vi "Reset.vi"(8 "error in (no error)":errorcluster, 11 "PWM in":refnum<class "LINX-PCA9685 PWM.lvclass">) -> (0 "error out":errorcluster, 3 "PWM out":refnum<class "LINX-PCA9685 PWM.lvclass">)   [LabVIEW 2020, in "LINX-PCA9685 PWM.lvclass"]
uses:
  LINX-PCA9685 PWM.lvclass
  LINX I2C/LINX I2C.lvclass
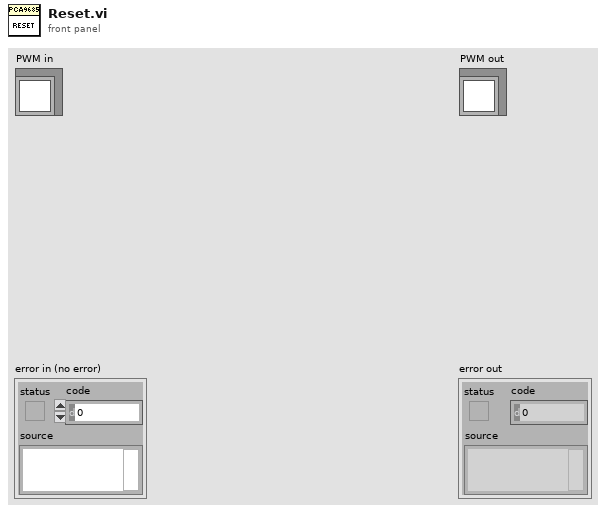
[diagram p1: front panel]
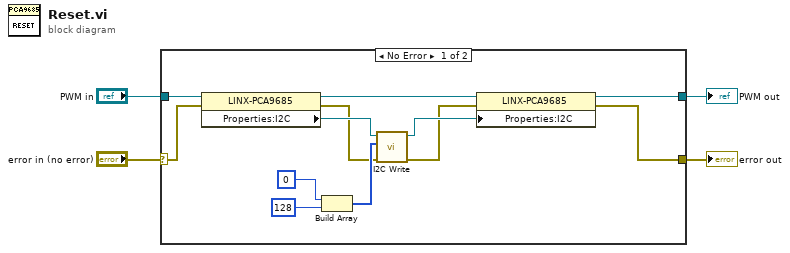
[diagram p0: block diagram]
diagram:
  n1 = case shown="No Error" "error in (no error)" {
    selector: "error in (no error)" -> [w6 w18]
    tunnel: [w7 w18] -> w3
    tunnel: [w9 w17] -> w1
    tunnel: "PWM in" -> [w13 w17]
    frame No Error {
      n2 = property class="LINX-PCA9685"(reference=w13, error in=w6) -> (reference out=w10:refnum<class "LINX-PCA9685 PWM.lvclass">, error out=w5:errorcluster, "Properties:I2C"=w12:refnum<class "LINX I2C.lvclass">)
      n3 = Build Array(u8 0 ("Address"), u8 128 ("Address")) -> (w16:u8[])
      n4 = call "I2C Write.vi"("error in (no error)"=w5, "Bytes to Write"=w16, "LINX I2C in"=w12) -> ("error out"=w8:errorcluster, "LINX I2C out"=w11:refnum<class "LINX I2C.lvclass">)  [unwired: 7 in]
      n5 = property class="LINX-PCA9685"(reference=w10, error in=w8, "Properties:I2C"=w11) -> (reference out=w9:refnum<class "LINX-PCA9685 PWM.lvclass">, error out=w7:errorcluster)
    }
    frame Error {
    }
  }
  "error out" <- w3
  "PWM out" <- w1
